vi "EventLogger.Init.vi"(5 "timestamp format":string="%c", 7 "Options":T1={"Max elements"=inf, "Max string length"=inf}, 8 "error in":errorcluster, 10 "Description":string, 11 "Path":path) -> (0 "error out":errorcluster, 3 "EventLog ref out":refnum<class "EventLog.lvclass">)   [LabVIEW 2019, in "Tools.lvlib"]
uses:
  Tools.lvlib
  <vilib>/NI/Event Logger Library/EventBuffer/Options.ctl
  <vilib>/NI/Event Logger Library/EventLog/EventLog.lvclass
  EventLogger.Manager.Action.ctl
  <vilib>/NI/Event Logger Library/EventLog/Initialize_CSV.vi
  <vilib>/NI/Event Logger Library/EventBuffer/EventBuffer.lvclass
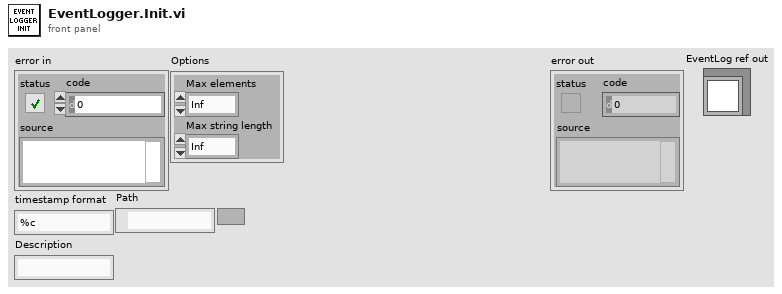
[diagram p1: front panel]
types:
  T1 = typedef "EventBuffer.lvclass/Options.ctl" = cluster{"Max elements":dbl, "Max string length":dbl}
  T2 = typedef "Tools.lvlib/EventLogger.Manager.Action.ctl" = enum16{"init", "get", "close"}
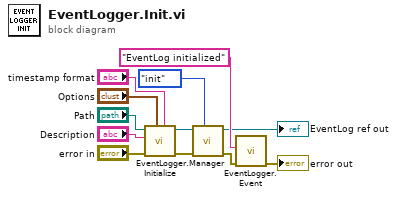
[diagram p0: block diagram]
diagram:
  n1 = call-poly <vilib>:"Initialize.vi"("timestamp format"="timestamp format", "Options"="Options", "error in (no error)"="error in", "Description"="Description", "Path"="Path") -> ("error out"=w12:errorcluster, "EventLog ref"=w5:refnum<class "EventLog.lvclass">)  [unwired: 5 in]
  n2 = call "EventLogger.Manager.vi"("action"=EventLogger.Manager.Action."init", "error in"=w12, "EventLog ref in"=w5) -> ("error out"=w3:errorcluster, "EventLog ref out"=→"EventLog ref out":refnum<class "EventLog.lvclass">)  [unwired: 7 in]
  n3 = call "EventLogger.Event.vi"("error in"=w3, "Event Name"="EventLog initialized") -> ("error out"=→"error out":errorcluster)  [unwired: 9 in]
